vi "Build Channel Acquisition String.vi"(8 "error in (no error)":errorcluster, 11 "5105 in":refnum<class "5105.lvclass">) -> (0 "error out":errorcluster, 2 "Channel Acquisition String":string, 3 "5105 out":refnum<class "5105.lvclass">)   [LabVIEW 2019, in "5105.lvlib" / "5105.lvclass"]
uses:
  5105.lvclass
  C:/Users/rdexter/Documents/Development/Drivers/PPL/Oscilloscope.lvlibp/Oscilloscope.lvclass
  builds/Instruments/Oscilloscope.lvlibp/Accessors/Read Channel Settings.vi
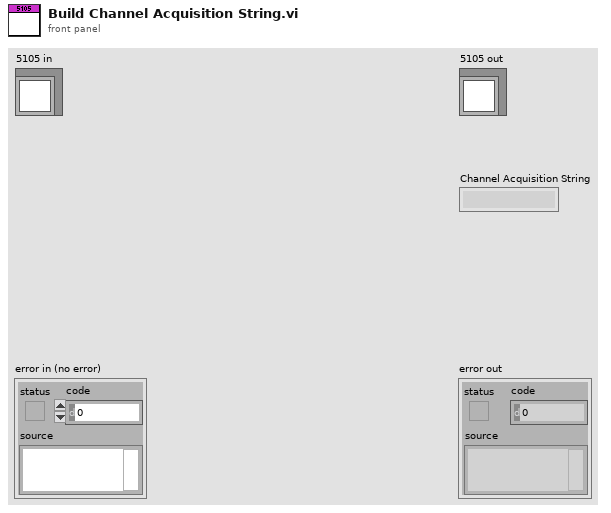
[diagram p1: front panel]
types:
  T1 = typedef "Oscilloscope.lvlibp/Oscilloscope.lvclass/Channel Settings.ctl" = cluster{"Amplitude":dbl, "Vertical Coupling":T2, "Probe Attenuation":dbl, "Enable?":bool, "Maximum Input Frequency":dbl, "Input Impedance":u16, "Timeout (s)":dbl}
  T2 = typedef "Oscilloscope.lvlibp/Oscilloscope.lvclass/Vertical Coupling.ctl" = enum16{"AC", "DC", "Ground"}
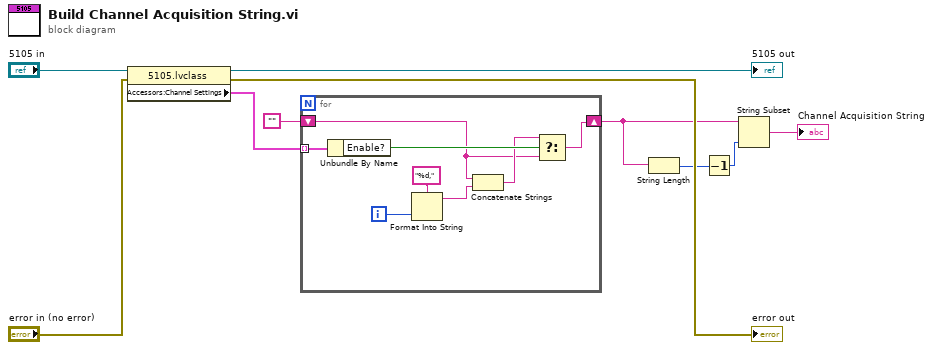
[diagram p0: block diagram]
diagram:
  n1 = property class="5105.lvclass"(reference="5105 in", error in="error in (no error)") -> (reference out=→"5105 out":refnum<class "5105.lvclass">, error out=→"error out":errorcluster, "Accessors:Channel Settings"=w8:T1[])
  n2 = for {
    tunnel: w8 -> [w18] mode=indexing
    shift-right: [w11] -> w2
    shift-left: "" -> [w12]
    i -> [w17]
    n3 = Unbundle By Name(w18) -> ("Enable?"=w14:bool)
    n4 = Format Into String(format string="%d,", w17) -> (resulting string=w15:string)  [unwired: 2 in, 1 out]
    n5 = Concatenate Strings(w12, w15) -> (w13:string)
    n6 = Select(t=w13, s=w14, f=w12) -> (s? t:f=w11:string)
  }
  n7 = String Length(string=w2) -> (length=w4:i32)
  n8 = Decrement(x=w4) -> (x-1=w1:i32)
  n9 = String Subset(string=w2, length (rest)=w1) -> (substring=→"Channel Acquisition String":string)  [unwired: 1 in]
